vi "Paul Lab2 Program.vi"() -> ()   [LabVIEW 2010]
uses:
  <vilib>/Utility/file.llb/Write To Spreadsheet File (DBL).vi
  <vilib>/Analysis/NI_AALBase.lvlib
panel:
  out "?":bool
  in  "Toggle to Save":bool
  in  "File Path":path
  out "XY Graph":T1(graph)
  in  "Histogram Intervals":i32
  out "Waveform Graph of random numbers":dbl[](graph)
  in  "Expected Value":dbl
  in  "Number of Random Numbers":i32
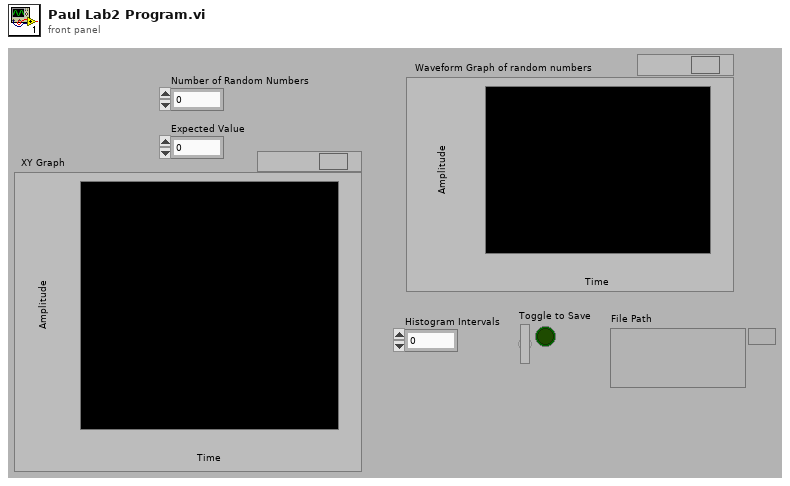
[diagram p1: front panel]
types:
  T1 = cluster{"X Values":dbl[], "Histogram: h(x)":i32[]}
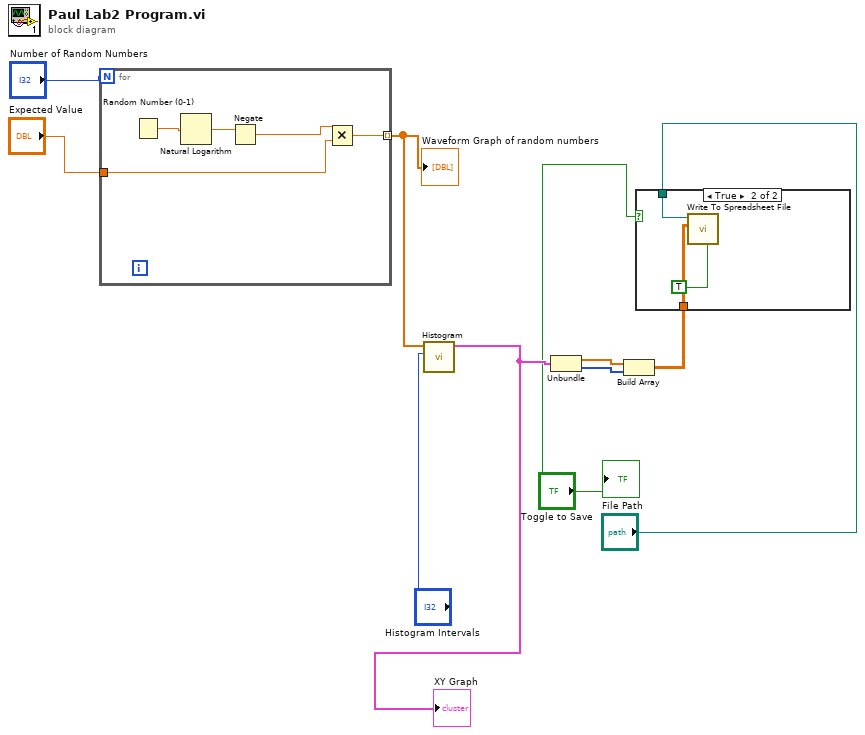
[diagram p0: block diagram]
diagram:
  n1 = for {
    N: "Number of Random Numbers" -> [_]
    tunnel: "Expected Value" -> [w12]
    tunnel: [w11] -> w7 mode=indexing
    n2 = Random Number (0-1)() -> (number: 0 to 1=w15:dbl)
    n3 = Natural Logarithm(1:w15) -> (0:w14:dbl)
    n4 = Negate(x=w14) -> (-x=w13:dbl)
    n5 = Multiply(x=w13, y=w12) -> (x*y=w11:dbl)
  }
  "Waveform Graph of random numbers" <- w7
  n6 = call <vilib>:"Histogram.vi"("intervals"="Histogram Intervals", "X"=w7) -> ("Histogram Graph"=w3:T1)  [unwired: 6 in, 3 out]
  "XY Graph" <- w3
  n7 = Unbundle(w3) -> ("X Values"=w6:dbl[], "Histogram: h(x)"=w5:i32[])
  n8 = Build Array(w6, w5) -> (w4:dbl[][])
  n9 = case shown="True" "Toggle to Save" {
    tunnel: w4 -> [_ w18]
    tunnel: "File Path" -> [_ w17]
    frame False {
    }
    frame True {
      n10 = call-poly <vilib>:"Write To Spreadsheet File.vi"("transpose? (no:F)"=TRUE, "2D data"=w18, "file path (dialog if empty)"=w17) -> ()  [unwired: 5 in, 1 out]
    }
  }
  "?" <- "Toggle to Save"
